vi "SynchronizeObjects.vi"(0 "connection ID":refnum<k5>, 2 "TargetClassInfo":T5(array[cluster]), 5 "error in (no error)":errorcluster, 6 "address":u32) -> (19 "error out":errorcluster)   [LabVIEW 2017, in "G#RemoteProxy.lvclass"]
doc: "Synchronizes the object cache."
uses:
  <vilib>/addons/_AddQ/G#Debugger/G#RemoteProxy/G#RemoteProxy.lvclass
  <vilib>/addons/_AddQ/G#Object/utils/G#Object_ClassInfoType.ctl
  <vilib>/addons/_AddQ/G#Object/utils/G#Object_ObjectInfoType.ctl
  <vilib>/addons/_AddQ/G#Object/utils/G#Object_CreateMethod.ctl
  <vilib>/addons/_AddQ/G#Object/G#Object.lvclass
  <vilib>/addons/_AddQ/G#Object/utils/G#Object_ClassHierarchy.ctl
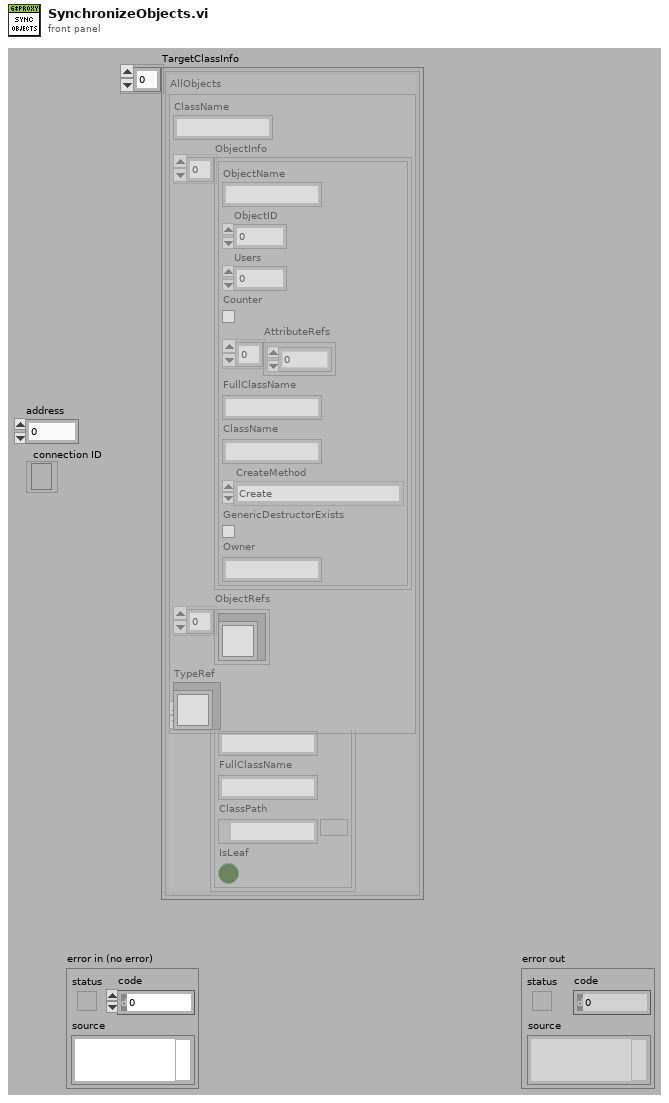
[diagram p1: front panel]
types:
  T1 = typedef "G#Object.lvclass/G#Object_ClassInfoType.ctl" = cluster{"ClassName":string, "ObjectInfo":T2[], "ObjectRefs":refnum<class "G#Object.lvclass">[], "TypeRef":refnum<class "G#Object.lvclass">}
  T2 = typedef "G#Object.lvclass/G#Object_ObjectInfoType.ctl" = cluster{"ObjectName":string, "ObjectID":u32, "Users":i32, "Counter":bool, "AttributeRefs":u32[], "FullClassName":string, "ClassName":string, "CreateMethod":T3, "GenericDestructorExists":bool, "Owner":string}
  T3 = typedef "G#Object.lvclass/G#Object_CreateMethod.ctl" = enum16{"Create", "Create or look up existing", "Look up existing"}
  T4 = typedef "G#Object.lvclass/G#Object_ClassHierarchy.ctl" = cluster{"ClassName":string, "FullClassName":string, "ClassPath":path, "IsLeaf":bool}
  T5 = cluster{"AllObjects":T1, "class hierarchy":T4[]}[]
  T6 = typedef "G#RemoteProxy.lvclass/ClassAttributesProxy.ctl" = cluster{"NoActiveProject":bool, "FullClassNames":string[], "FullClassPaths":path[], "RemoteRefs":refnum<class "G#Object.lvclass">[], "ProxyRefs":refnum<class "G#RemoteProxy.lvclass">[], "RemoteClassName":string[], "ProxyClassRefs":refnum<class "G#RemoteProxy.lvclass">[]}
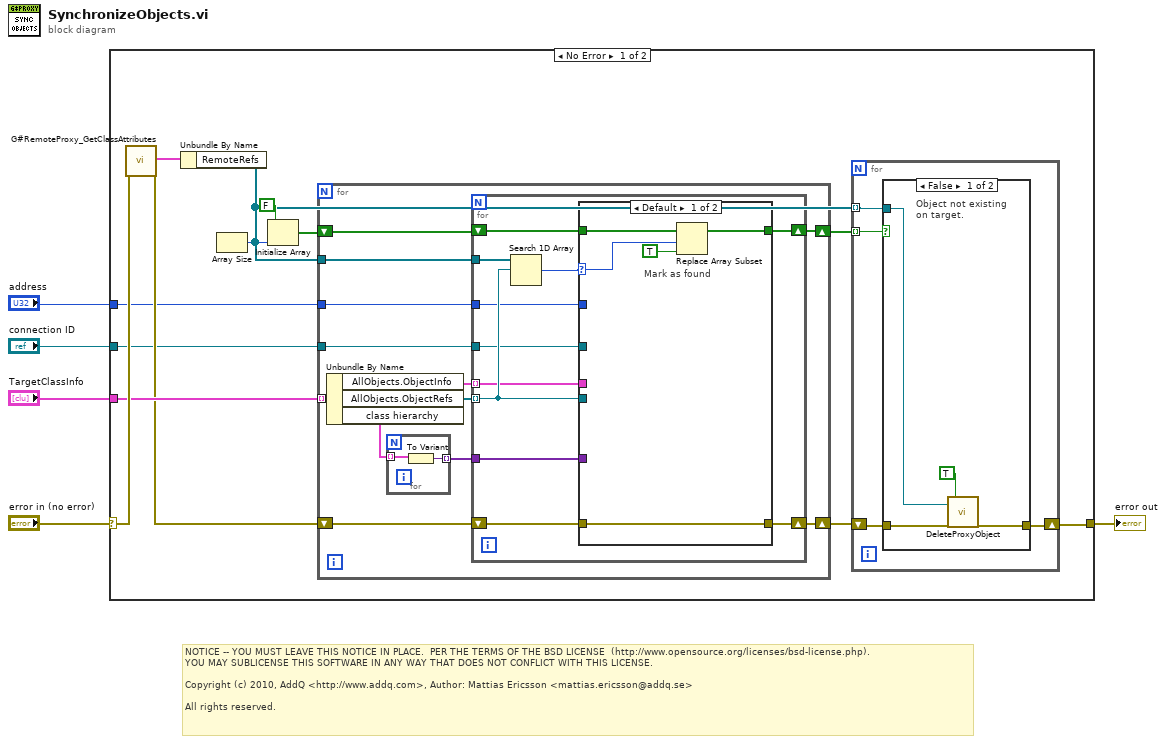
[diagram p0: block diagram]
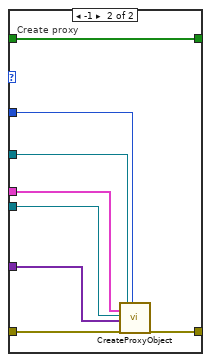
[diagram p3: hidden frame]
diagram:
  # "NOTICE -- YOU MUST LEAVE THIS NOTICE IN PLACE.  PER THE TERMS OF THE BSD LICENSE  (http://www.opensource.org/licenses/bsd-license.php).\nYOU MAY SUBLICENSE THIS SOFTWARE IN ANY WAY THAT DOES NOT CONFLICT WITH THIS LICENSE.\n\nCopyright (c) 2010, AddQ <http://www.addq.com>, Author: Mattias Ericsson <mattias.ericsson@addq.se>\n\nAll rights reserved."
  n1 = case shown="No Error" "error in (no error)" {
    selector: "error in (no error)" -> [w18 w66]
    tunnel: [w8 w66] -> w4
    tunnel: "TargetClassInfo" -> [w17 _]
    tunnel: "connection ID" -> [w7 _]
    tunnel: "address" -> [w6 _]
    frame No Error {
      n2 = call <vilib>:"G#RemoteProxy_GetClassAttributes.vi"("error in (no error)"=w18) -> ("class attributes"=w16:T6, "error out"=w15:errorcluster)  [unwired: 15 in, 2 out]
      n3 = Unbundle By Name(w16) -> ("RemoteRefs"=w10:refnum<class "G#Object.lvclass">[])
      n4 = Array Size(array=w10) -> (size(s)=w13:i32)
      n5 = Initialize Array(FALSE, w13) -> (w14:bool[])
      n6 = for {
        tunnel: w17 -> [w39] mode=indexing
        shift-right: [w34] -> w11
        shift-left: w15 -> [w37]
        shift-right: [w33] -> w9
        shift-left: w14 -> [w36]
        tunnel: w10 -> [w32]
        tunnel: w7 -> [w29]
        tunnel: w6 -> [w28]
        n7 = Unbundle By Name(w39) -> ("AllObjects.ObjectInfo"=w35:T2[], "AllObjects.ObjectRefs"=w38:refnum<class "G#Object.lvclass">[], "class hierarchy"=w31:T4[])
        n8 = for {
          tunnel: w31 -> [w41] mode=indexing
          tunnel: [w40] -> w30 mode=indexing
          n9 = To Variant(anything=w41) -> (Variant=w40:variant)
        }
        n10 = for {
          tunnel: w32 -> [w52]
          tunnel: w38 -> [w46] mode=indexing
          shift-right: [w48] -> w34
          shift-left: w37 -> [w47]
          shift-right: [w49] -> w33
          shift-left: w36 -> [w50]
          tunnel: w35 -> [w45] mode=indexing
          tunnel: w30 -> [w44]
          tunnel: w29 -> [w43]
          tunnel: w28 -> [w42]
          n11 = Search 1D Array(1D array=w52, element=w46) -> (index of element=w51:i32)  [unwired: 1 in]
          n12 = case shown="Default" w51 {
            selector: w51 -> [w55 _]
            tunnel: w50 -> [w57 w65]
            tunnel: [w56 w65] -> w49
            tunnel: [w53 w64] -> w48
            tunnel: w47 -> [w53 w63]
            tunnel: w46 -> [_ w62]
            tunnel: w45 -> [_ w61]
            tunnel: w44 -> [_ w60]
            tunnel: w43 -> [_ w59]
            tunnel: w42 -> [_ w58]
            frame Default {
              # "Mark as found"
              n13 = Replace Array Subset(array=w57, new element=TRUE ("new element/subarray"), index=w55) -> (w56:bool[])
            }
            frame -1 {
              # "Create proxy"
              n14 = call <vilib>:"CreateProxyObject.vi"("object info"=w61, "remote object ref"=w62, "parameters"=w60, "error in (no error)"=w63, "connection ID"=w59, "address"=w58) -> ("error out"=w64:errorcluster)  [unwired: 13 in]
            }
          }
        }
      }
      n15 = for {
        shift-right: [w20] -> w8
        shift-left: w11 -> [w21]
        tunnel: w10 -> [w19] mode=indexing
        tunnel: w9 -> [w22] mode=indexing
        n16 = case shown="False" w22 {
          tunnel: w21 -> [w26 w27]
          tunnel: [w25 w27] -> w20
          tunnel: w19 -> [w23 _]
          frame False {
            # "Object not existing\non target."
            n17 = call <vilib>:"DeleteProxyObject.vi"("remote object ref"=w23, "error in (no error)"=w26, "force delete? (F)"=TRUE) -> ("error out"=w25:errorcluster)  [unwired: 16 in]
          }
          frame True {
          }
        }
      }
    }
    frame Error {
    }
  }
  "error out" <- w4
